vi "HTTP_POST_TEST02.vi"() -> ()   [LabVIEW 2018]
uses:
  <vilib>/httpClient/POSTBuffer.vi
  <vilib>/httpClient/LabVIEWHTTPClient.lvlib
panel:
  out "Web":string="http://ricky10116.pythonanywhere.com/index.html"
  out "Result":string
  out "Title":string="LabVIEW and Http POST"
  in  "ReadHTML":bool
  in  "Stop Button":bool
  in  "POST Button":bool
  in  "Test1":string
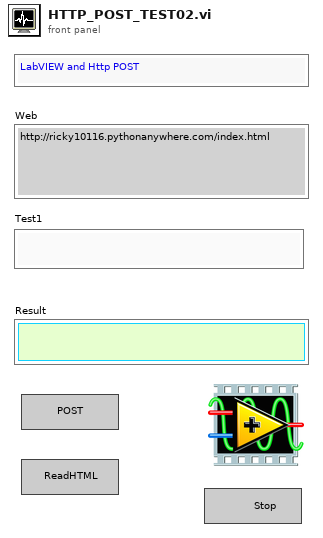
[diagram p1: front panel]
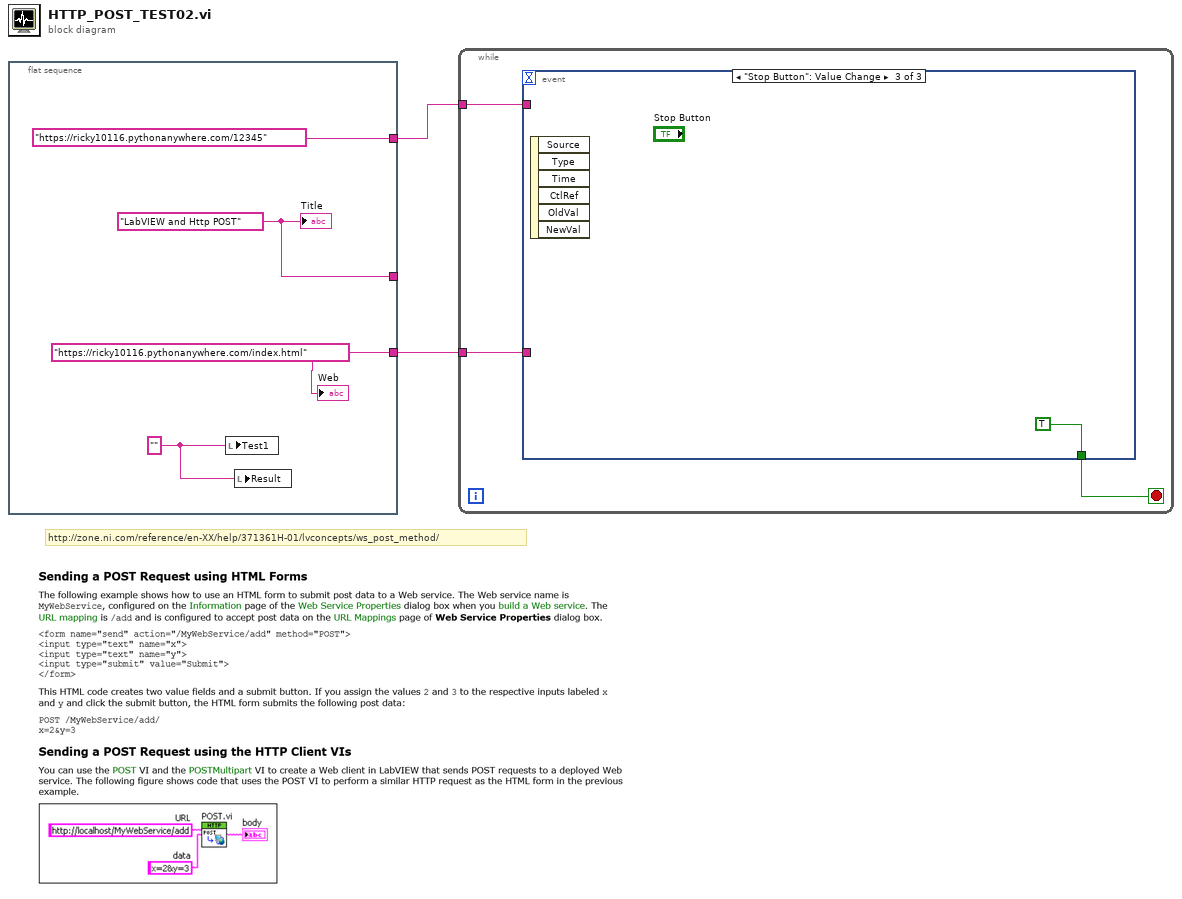
[diagram p0: block diagram]
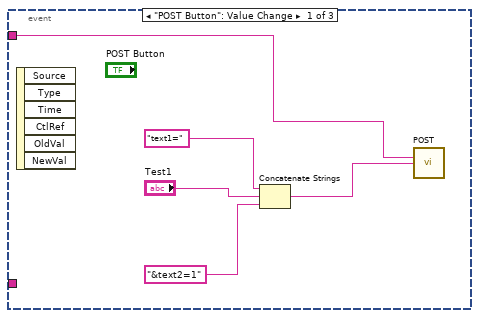
[diagram p2: hidden frame]
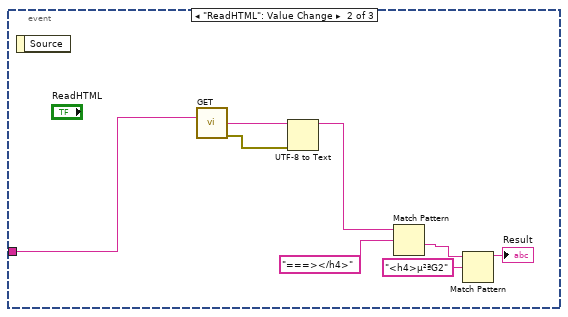
[diagram p3: hidden frame]
diagram:
  # "http://zone.ni.com/reference/en-XX/help/371361H-01/lvconcepts/ws_post_method/"
  n1 = flat-sequence {
    tunnel: [w6] -> _
    tunnel: ["https://ricky10116.pythonanywhere.com/12345" ("url")] -> w2
    tunnel: [w3] -> w1
    frame #0 {
      w4 = "" ("Test1")
      w3 = "https://ricky10116.pythonanywhere.com/index.html"
      w6 = "LabVIEW and Http POST" ("Title")
      n2 = local write "Test1"(w4) -> ()
      n3 = local write "Result"(w4) -> ()
      "Title" <- w6
      "Web" <- w3
    }
  }
  n4 = while {
    tunnel: w2 -> [w8]
    tunnel: w1 -> [w7]
    stop <- w9 stop-if-true
    n5 = event shown="[2] \"Stop Button\": Value Change" {
      selector: _ -> [_ _ _]
      dyn-events: _ -> [_ _ _]
      timeout: _ -> [_ _ _]
      tunnel: [_ _ TRUE] -> w9
      tunnel: w8 -> [w10 _ _]
      tunnel: w7 -> [_ w20 _]
      event "POST Button": Value Change {
        n6 = event-data() -> ()  [unwired: 1 in, 6 out]
        n7 = Concatenate Strings("text1=", "Test1", "&text2=1") -> (w11:string)
        n8 = call-poly <vilib>:"POST.vi"("url"=w10, "buffer"=w11) -> ()  [unwired: 10 in, 4 out]
      }
      event "ReadHTML": Value Change {
        n9 = event-data() -> ()  [unwired: 1 in, 1 out]
        n10 = call <vilib>:"GET.vi"("url"=w20) -> ("body"=w22:string, "error out"=w21:errorcluster)  [unwired: 11 in, 2 out]
        n11 = UTF-8 to Text(8:w21, 11:w22) -> (3:w19:string)  [unwired: 1 in, 1 out]
        n12 = Match Pattern(string=w19, regular expression="===></h4>") -> (after substring=w17:string)  [unwired: 1 in, 3 out]
        n13 = Match Pattern(string=w17, regular expression="<h4>µ²ªG2") -> (before substring=→"Result":string)  [unwired: 1 in, 3 out]
      }
      event "Stop Button": Value Change {
        n14 = event-data() -> ()  [unwired: 1 in, 6 out]
      }
    }
  }
